vi "readTriggering.vi"(8 "error in (no error)":errorcluster, 10 "triggering":string, 11 "FileReader in":refnum<class "FileReader.lvclass">) -> (0 "error out":errorcluster, 1 "start trigger line":string, 2 "clock source":string, 3 "FileReader out":refnum<class "FileReader.lvclass">)   [LabVIEW 2011, in "Tools.lvlib" / "Filing.lvlib" / "FileReader.lvclass"]
uses:
  FileReader.lvclass
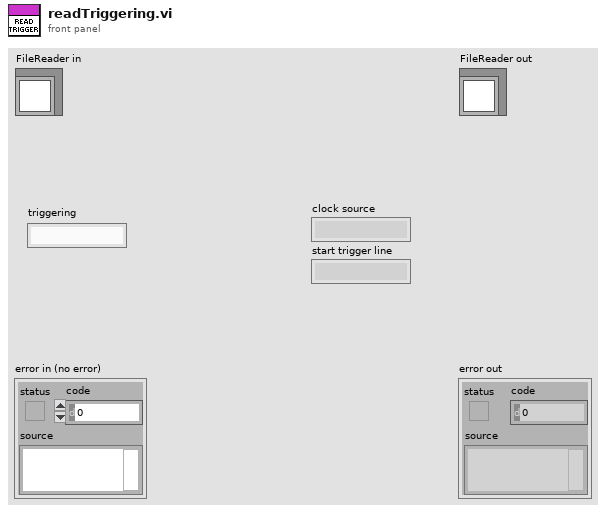
[diagram p1: front panel]
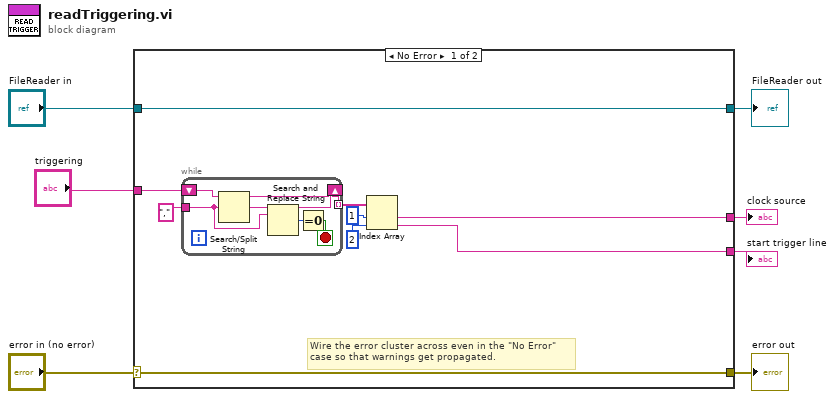
[diagram p0: block diagram]
diagram:
  n1 = case shown="No Error" "error in (no error)" {
    selector: "error in (no error)" -> [w15 w25]
    tunnel: [w15 w25] -> w6
    tunnel: [w16 w24] -> w4
    tunnel: "FileReader in" -> [w16 w24]
    tunnel: "triggering" -> [w11 _]
    tunnel: [w9 _] -> w2
    tunnel: [w8 _] -> w1
    frame No Error {
      # "Wire the error cluster across even in the \"No Error\"\ncase so that warnings get propagated."
      n2 = while {
        tunnel: "," ("search string/char (-)") -> [w21]
        shift-right: [w19] -> _
        shift-left: w11 -> [w23]
        tunnel: [w17] -> w14 mode=indexing
        stop <- w20 stop-if-true
        n3 = Search/Split String(string=w23, search string/char (-)=w21) -> (substring before match=w17:string, match + rest of string=w22:string)  [unwired: 1 in, 1 out]
        n4 = Search and Replace String(input string=w22, search string=w21) -> (result string=w19:string, number of replacements=w18:i32)  [unwired: 6 in, 2 out]
        n5 = Equal To 0?(x=w18) -> (x = 0?=w20:bool)
      }
      n6 = Index Array(array=w14, index #1=1 ("index"), index #2=2 ("index")) -> (element #1=w9:string, element #2=w8:string)
    }
    frame Error {
    }
  }
  "error out" <- w6
  "FileReader out" <- w4
  "clock source" <- w2
  "start trigger line" <- w1
